vi "Trauma Box Controller.vi"() -> ()   [LabVIEW 2020]
uses:
  epl-vi-lib/Utility VIs/Buttons/KCheckmarkBoolean.ctl
  epl-vi-lib/Utility VIs/Controls/KBackground Gradient/KBackground Gradient.xctl
  Typedefs/TB-Parameters.ctl
  epl-vi-lib/Signal Synthesis VIs/Controls/Waveform XCtl/Waveform Enum.ctl
  Typedefs/TB-Slack State.ctl
  Typedefs/TB-State Enum.ctl
  <vilib>/Analysis/baseanly.llb/Mean (DBL).vi
  <vilib>/Analysis/5stat.llb/RMS (DBL).vi
  epl-vi-lib/Utility VIs/Math VIs/Linear to dB (scalar).vi
  epl-vi-lib/Connection VIs/Connection Manager.vi
  <vilib>/Analysis/NI_AALPro.lvlib
  <vilib>/Analysis/NI_AALBase.lvlib
  <vilib>/gmath/NI_Gmath.lvlib
panel:
  out "Exposure":errorcluster
  out "Crown":errorcluster
  in  "Waveform":u16(ring)=2 items=["Noise"=2, "File"=4, "Tone"=1]
  in  "dB SPL":dbl=100.0
  in  "Duration (min)":dbl=120.0
  in  "Tab Control":enum32{"Tone", "Noise", "File"}(tab)
  in  "Frequency (kHz)":dbl=8.0
  in  "High cutoff (kHz)":dbl=16.0
  in  "Low cutoff (kHz)":dbl=8.0
  in  "refWAV":path caption="Ref"
  in  "WAVfile":path
  in  "Cal Log":path=path "C:/Data/Trauma Box/Trauma Box Calibration Log.txt"
  out "Pistonphone Factor":dbl=102.0 caption="Calibrator Voltage\n(dB rms re 1 uV)"
  in  "B&K Mic Gain":dbl=20.0
  in  "Display":enum32{"Page 1", "Page 2"}(tab)
  out "ma":dbl=99.37258874088361 caption="average" format="%.1f"
  out "Starts":i32
  out "Overload 2":bool caption="Overload"
  in  "Fine Control":dbl(slide) caption="Fine Adjust (dB)" scale=0.0..1.0
  out "Spectrum":waveform(dbl)(graph)
  out "Waveform":waveform(dbl)(graph)
  out "dB SPL rms":dbl=99.37258874088361 format="%.2f"
  out "Gauge":dbl(knob)=99.37258874088361 scale=80.0..130.0
  out "Elapsed time":string
  out "SPL History":cluster{dbl[], dbl[]}[](graph)
  out "Expected":string="Expected value = 102"
  in  "micCorrFile":path
  in  "Use mic correction":T1 caption="Apply mic frequency correction (if you're unsure, then no)"
  out "Calibration Log":string[][](table)
  out "Overload":bool
  out "Calibrator Voltage\n(dB rms re 1 uV)":dbl=-inf
  out "Pistonphone\nWaveform":dbl[](graph)
  in  "Wizard":T2(tab)
  in  "START":bool
  in  "EXIT":bool
  in  "Use previous":bool
  in  "Remeasure":bool
  in  "Pistonphone measure":bool
  in  "Next":bool
  in  "To Crown adjust":bool
  in  "Start Crown":bool
  in  "Stop Crown":bool
  in  "Start Trauma":bool
  in  "Stop Trauma":bool
  in  "Finished":bool
  in  "User ID":string
  in  "Gradient":dbl(xcontrol)
  # "dB SPL"
  # "Press START to begin\nPress EXIT to quit"
  # "Step 1 Pistonphone correction"
  # "Step 1 Pistonphone correction\n    \n--Put ref mic into pistonphone\n--Make sure B&K gain is correct"
  # "Step 2 Put microphone in cage. It's going to get loud! Close the booth door before continuing."
  # "Step 3 Adjust amplifier until SPL is correct, then hit \"Stop\" button:"
  # "Step 4: Noise Exposure\n1. Put animal(s) in cage\n2. Set duration,\n3. Press START"
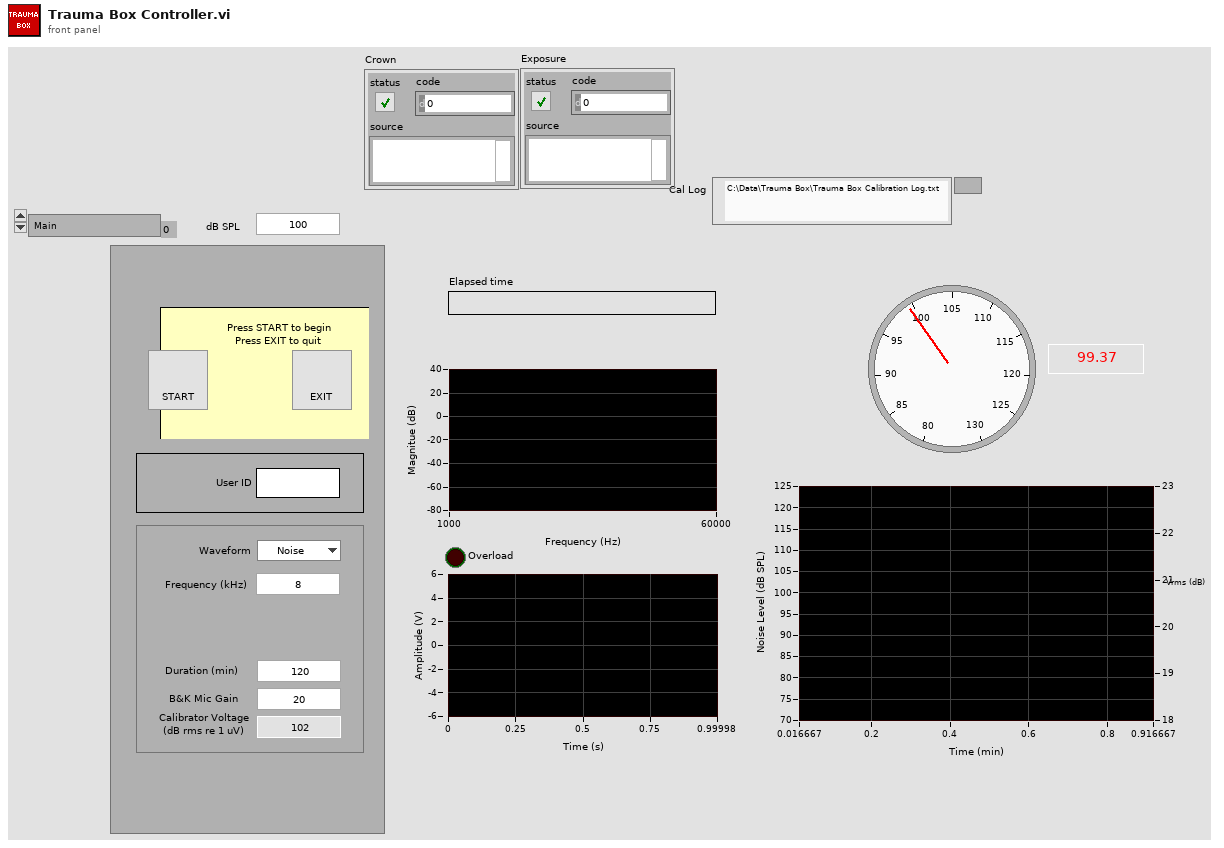
[diagram p1: front panel]
types:
  T1 = typedef "KCheckmarkBoolean.ctl" = bool
  T2 = enum32{"Main", "Pistonphone query", "Pistonphone measure", "Mic in cage", "Adjust Crown", "Animal in cage"}
  T3 = typedef "TB-Parameters.ctl" = cluster{"Low cutoff (kHz)":dbl, "High cutoff (kHz)":dbl, "Duration (min)":dbl, "dB SPL":dbl, "Waveform":T4, "WAVfile":path, "refWav":path, "use mic correction":bool, "micCorrFile":path, "Pistonphone Level (dB SPL)":dbl, "Sampling rate (Hz)":dbl, "Buffer length (s)":dbl, "Stream mic":bool, "Fine adjust":cluster{"Max":dbl, "Min":dbl}, "Mic gain":dbl, "atten":dbl, "resol (Hz)":dbl, "navgs":i32, "Allow Slack":bool, "max starts":i32, "Freq (kHz)":dbl, "Tma (s)":dbl, "Streamed":cluster{"Num":i32, "Name":string}[], "Drive":string}
  T4 = typedef "Waveform Enum.ctl" = enum16{"OFF", "Tone", "Noise", "Pulse Train", "File", "FM Sweep", "Chirp Train", "Complex Tone", "FM Tone", "Moving Ripple"}
  T5 = typedef "TB-Slack State.ctl" = cluster{"access_token":string, "bot id":string, "users":cluster{"id":string, "always":bool}[], "chan id":string}
  T6 = cluster{bool, "Exposure parameters":T3, "Slack":T5}
  T7 = typedef "TB-State Enum.ctl" = enum16{"Main", "Pistonphone query", "Pistonphone measure", "Mic in cage", "Adjust Crown", "Animal in cage"}
  T8 = enum16{"arithmetic", "geometric", "harmonic", "trimmed", "median"}
  T9 = cluster{"notification":bool, "Exposure parameters":T3, "Slack":T5}
  T10 = typedef "TB-Runtime state.ctl" = cluster{"stimfile":T11, "stream mic?":bool, "Fs":dbl, "ID":string, "micCorr":dbl[], "navg":i32, "r2sum":dbl[], "expose":bool, "spectra/frame":i32, "pts/spectra":i32, "nacq":i32, "init error":bool, "max starts":i32, "num starts":i32, "Setup":T12, "toneIndex":i32, "LastN":dbl[], "fine":dbl, "imic":i32, "stream":refnum<file>, "names":string[]}
  T11 = typedef "Sound File Refnum.ctl" = refnum<file>
  T12 = typedef "TB-Setup Log.ctl" = cluster{"Pistonphone factor":dbl, "Fine adjust":dbl, "Actual dB SPL":dbl, "Freq":dbl[], "Mag":dbl[]}
  T13 = typedef "TB-Stimulus State.ctl" = cluster{"filelen":i32, "stimfile":T11, "stimfile?":bool, "Fs":dbl, "Npts":i32, "stimfileend":bool, "atten":dbl, "AO":i32[]}
  T14 = typedef "Waveform XCtl.xctl/Waveform Data.ctl" = cluster{"Type":T4, "Tone":T15, "Pulse Train":T16, "Noise":T19, "File":T20, "FMSweep":T21, "Chirp Train":T22, "Complex Tone":cluster{"Params":T24, "Data":T26}, "Moving Ripple":T27}
  T15 = typedef "Tone Params.ctl" = cluster{"Frequency (kHz)":dbl, "Last Freq":dbl, "Last Phase":dbl}
  T16 = typedef "Pulse Train Params.ctl" = cluster{"Pulse width (us)":dbl, "Pulse rate (Hz)":dbl, "Gap (ms)":dbl, "Polarity":T17, "PT State":T18, "Asynch":bool}
  T17 = typedef "Pulse Polarity.ctl" = enum16{"POS", "NEG", "POS-NEG", "NEG-POS"}
  T18 = typedef "PT-Continuous State.ctl" = cluster{"Template":dbl[], "Nperiod":i32, "Index":i32, "Pulse Rate (Hz)":dbl, "Phase (cycles)":dbl, "Noff":i32}
  T19 = typedef "Noise Params.ctl" = cluster{"InvFilt":bool, "Noise":dbl[], "CurPt":i32, "Aweight":bool, "Seed":i32, "afile":path}
  T20 = typedef "StimFile-Params.ctl" = cluster{"Filename":path, "Signal":dbl[], "Channel":i32, "stream":bool, "offset":i32, "nreps":i32, "loops":i32, "Randomize":bool, "order":i32[], "Seed":i32, "Tokens":i32}
  T21 = typedef "FM Sweep Params.ctl" = cluster{"Rate (oct/s)":dbl, "Fmin (Hz)":dbl, "Fmax (Hz)":dbl, "Ramp (ms)":dbl, "Linear":bool}
  T22 = typedef "Chirp Train.ctl" = cluster{"Params":T23, "Data":cluster{"WF":dbl[]}}
  T23 = typedef "Chirp Train Params.ctl" = cluster{"Fmin (kHz)":dbl, "Fmax (kHz)":dbl, "Compensate":bool, "Duration (ms)":dbl}
  T24 = typedef "CT-Params.ctl" = cluster{"F0 (Hz)":dbl, "Band":cluster{"Flow (Hz)":dbl, "Fhigh (Hz)":dbl}, "Phase":T25, "Min F0 (Hz)":dbl, "Max F0 (Hz)":dbl, "ContinRandPhase":bool, "Max peak factor":dbl, "Max mod depth":dbl, "MinHarmNum":i32, "MaxHarmNum":i32, "Level Mode":enum16{"per component", "overall rms"}, "% jitter":dbl}
  T25 = typedef "CT-Phase Enum.ctl" = enum16{"Cosine", "Random", "Alternating"}
  T26 = typedef "CT-Runtime Data.ctl" = cluster{"Ncomp":i32, "MinHarm":i32, "Phase":dbl[], "Amplitude":dbl[], "Npts/frame":i32, "Last F0":dbl, "Fmin":dbl, "Fmax":dbl, "Lslope":dbl, "randphase":bool, "overall rms":bool, "fmult":dbl[], "jittered":bool}
  T27 = typedef "Moving Ripple.ctl" = cluster{"Params":T28, "Data":T29}
  T28 = typedef "Moving Ripple.Params.ctl" = cluster{"Fmin":dbl, "Fmax":dbl, "Density":dbl, "Velocity":dbl, "Depth":dbl, "Phase":dbl, "Comp/oct":i32}
  T29 = typedef "Moving Ripple.Data.ctl" = cluster{"Freq":dbl[], "A":dbl[], "phase":dbl[], "Phase":dbl}
  T30 = typedef "Filter XCtl.xctl/Filter Data.ctl" = cluster{"CF (kHz)":dbl, "BW (kHz)":dbl, "IIR Filter Cluster":cluster{"filter structure":enum32{"IIR 2nd Order", "IIR 4th Order"}, "Reverse Coefficients":dbl[], "Forward Coefficients":dbl[]}, "Final Filter State":dbl[], "Scale Factor":dbl, "Final Filter State 2":dbl[], "Quadrature":bool, "Type":enum16{"Lowpass", "Highpass", "Bandpass", "Bandstop", "OFF"}}
  T31 = typedef "Gate Control.xctl/Gate Data.ctl" = cluster{"Active":bool, "Delay (ms)":dbl, "Width (ms)":dbl, "Ramp (ms)":dbl}
  T32 = typedef "Level XCtl.xctl/Level Data.ctl" = cluster{"Level":dbl, "Units":T33, "Max":dbl, "Multiplier":dbl, "Cal File":path, "Cal":cluster{"Freq (Hz)":dbl[], "Mag (dB SPL)":dbl[], "Phase (deg)":dbl[]}}
  T33 = typedef "Level Units.ctl" = enum16{"dB atten", "dB SPL", "dB re 1 Vrms", "dB V/Hz½", "mW", "dB HL", "Volts", "dB mW"}
  T34 = cluster{"Waveform":T14, "Filter":T30, "Gate":T31, "Level":T32}
  T35 = typedef "TB-Log.ctl" = cluster{"Slack":T5, "entries":string[]}
  T36 = typedef "TB-Mic Queue.ctl" = refnum<queue>
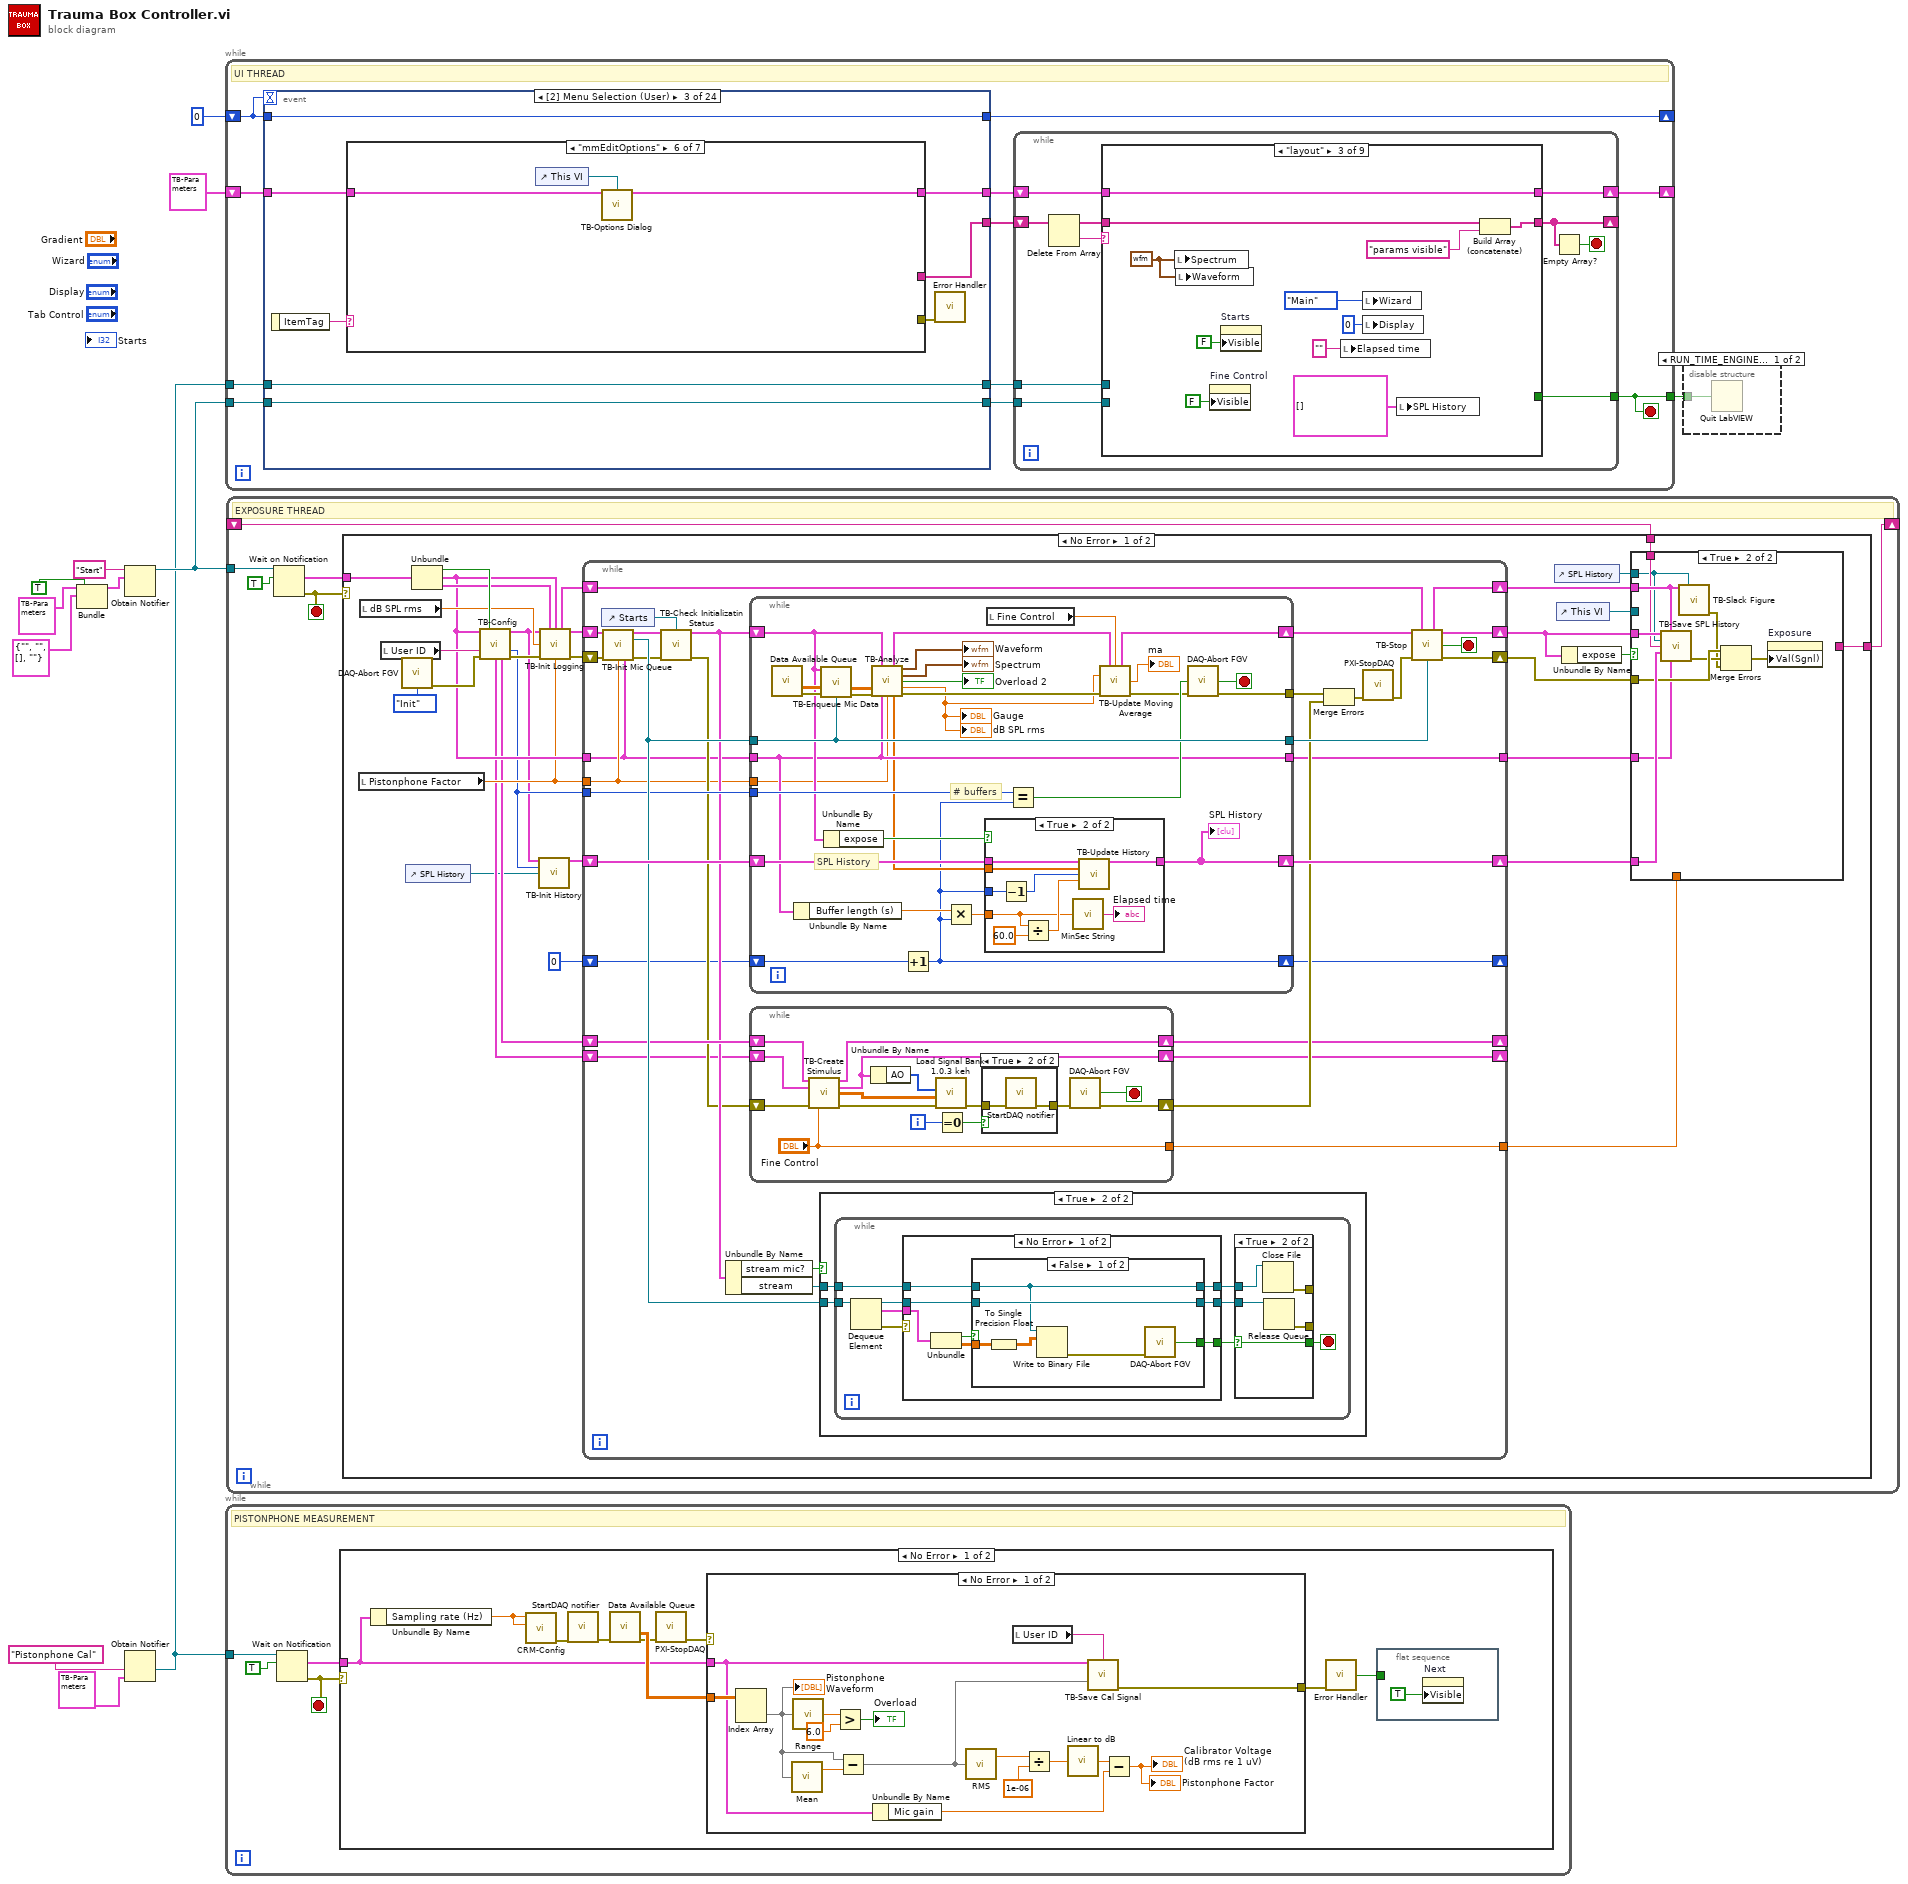
[diagram p0: block diagram]
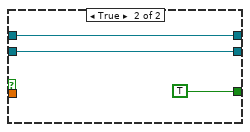
[diagram p6: hidden frame]
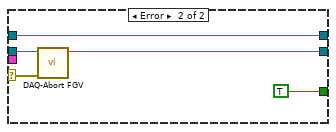
[diagram p7: hidden frame]
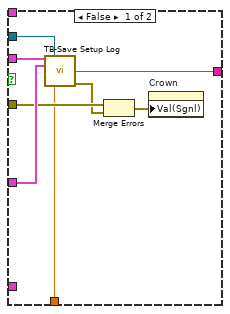
[diagram p8: hidden frame]
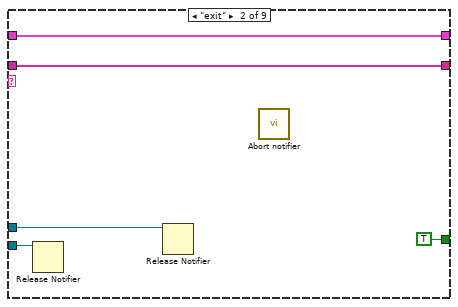
[diagram p11: hidden frame]
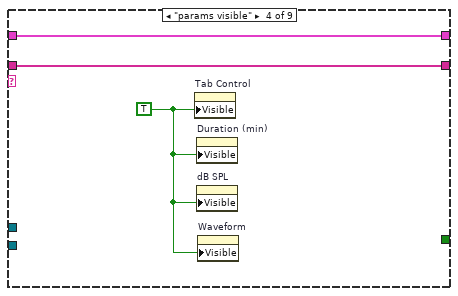
[diagram p12: hidden frame]
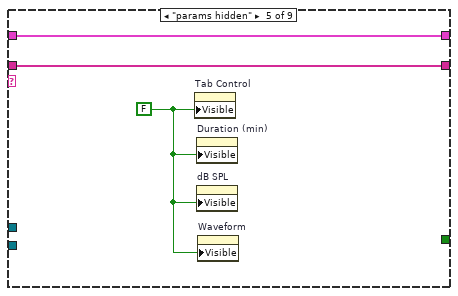
[diagram p13: hidden frame]
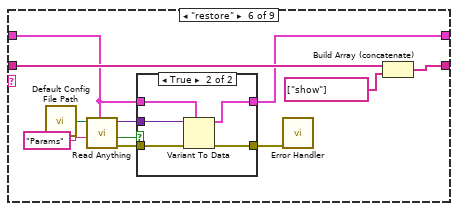
[diagram p14: hidden frame]
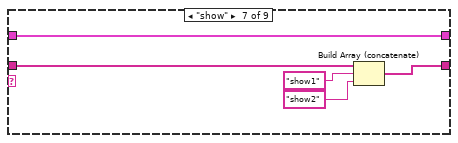
[diagram p16: hidden frame]
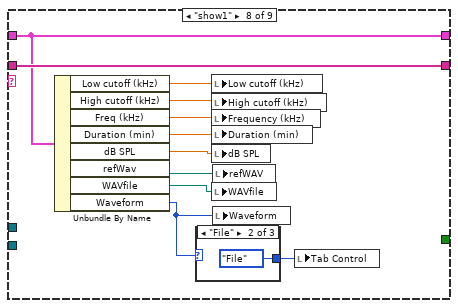
[diagram p17: hidden frame]
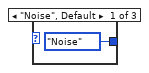
[diagram p18: hidden frame]
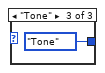
[diagram p19: hidden frame]
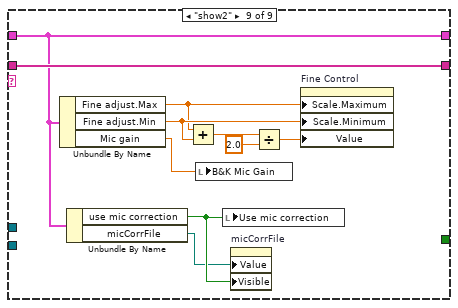
[diagram p20: hidden frame]
diagram:
  n1 = Bundle(TRUE, "Exposure parameters"=T3 {"Low cutoff (kHz)"=0.0, "High cutoff (kHz)"=0.0, "Duration (min)"=0.0, "dB SPL"=0.0, "Waveform"=enum."OFF", "WAVfile"=path "", "refWav"=path "", "use mic correction"=FALSE, "micCorrFile"=path "", "Pistonphone Level (dB SPL)"=0.0, "Sampling rate (Hz)"=0.0, "Buffer length (s)"=0.0, "Stream mic"=FALSE, "Fine adjust"={"Max"=0.0, "Min"=0.0}, "Mic gain"=0.0, "atten"=0.0, "resol (Hz)"=0.0, "navgs"=0, "Allow Slack"=FALSE, "max starts"=0, "Freq (kHz)"=8.0, "Tma (s)"=0.0, "Streamed"=[], "Drive"=""}, "Slack"=T5 {"access_token"="", "bot id"="", "users"=[], "chan id"=""}) -> (w4:T6)  [unwired: 1 in]
  n2 = Obtain Notifier(name (unnamed)="Start", notification data type=w4) -> (notifier out=w12:refnum<notifier>)  [unwired: 2 in, 2 out]
  n3 = Obtain Notifier(name (unnamed)="Pistonphone Cal", notification data type=T3 {"Low cutoff (kHz)"=114.0, "High cutoff (kHz)"=100000.0, "Duration (min)"=1.0, "dB SPL"=100.0, "Waveform"=enum."Noise", "WAVfile"=path "", "refWav"=path "", "use mic correction"=FALSE, "micCorrFile"=path "", "Pistonphone Level (dB SPL)"=0.0, "Sampling rate (Hz)"=0.0, "Buffer length (s)"=0.0, "Stream mic"=FALSE, "Fine adjust"={"Max"=0.0, "Min"=0.0}, "Mic gain"=0.0, "atten"=0.0, "resol (Hz)"=0.0, "navgs"=0, "Allow Slack"=FALSE, "max starts"=0, "Freq (kHz)"=8.0, "Tma (s)"=0.0, "Streamed"=[], "Drive"=""} ("Exposure parameters")) -> (notifier out=w8:refnum<notifier>)  [unwired: 2 in, 2 out]
  n4 = while {
    tunnel: w12 -> [w23]
    shift-right: [w22] -> _
    shift-left: 0 -> [w19]
    tunnel: w8 -> [w21]
    tunnel: [w13] -> w7
    shift-right: [w14] -> _
    shift-left: T3 {"Low cutoff (kHz)"=8.0, "High cutoff (kHz)"=16.0, "Duration (min)"=120.0, "dB SPL"=100.0, "Waveform"=enum."Noise", "WAVfile"=path "", "refWav"=path "", "use mic correction"=FALSE, "micCorrFile"=path "", "Pistonphone Level (dB SPL)"=114.0, "Sampling rate (Hz)"=100000.0, "Buffer length (s)"=1.0, "Stream mic"=FALSE, "Fine adjust"={"Max"=0.0, "Min"=0.0}, "Mic gain"=0.0, "atten"=0.0, "resol (Hz)"=0.0, "navgs"=0, "Allow Slack"=FALSE, "max starts"=3, "Freq (kHz)"=8.0, "Tma (s)"=0.0, "Streamed"=[], "Drive"=""} ("Exposure parameters") -> [w20]
    stop <- w13 stop-if-true
    # "UI THREAD"
    n5 = event shown="[2] Menu Selection (User)" {
      selector: _ -> [_ _ _ _ _ _ _ _ _ _ _ _ _ _ _ _ _ _ _ _ _ _ _ _]
      dyn-events: _ -> [_ _ _ _ _ _ _ _ _ _ _ _ _ _ _ _ _ _ _ _ _ _ _ _]
      timeout: w19 -> [_ _ _ _ _ _ _ _ _ _ _ _ _ _ _ _ _ _ _ _ _ _ _ _]
      tunnel: w23 -> [_ w139 w146 _ _ _ _ _ _ _ _ _ _ _ _ w248 w256 _ w291 _ _ w312 _ _]
      tunnel: [_ w139 w146 _ _ _ _ _ _ _ _ _ _ _ _ _ _ _ _ _ _ w312 _ _] -> w16
      tunnel: [-1 w142 w150 w178 w184 w190 w193 w198 w206 w207 w212 w219 w223 w229 w232 w241 w252 w264 w274 w303 w305 w309 w316 w320] -> w22
      tunnel: w21 -> [_ w140 w147 _ _ _ _ _ _ _ _ _ _ w230 _ _ _ _ _ _ _ w311 _ _]
      tunnel: [_ w140 w147 _ _ _ _ _ _ _ _ _ _ _ _ _ _ _ _ _ _ w311 _ _] -> w17
      tunnel: [w109 w143 w148 w179 w187 w191 w196 w201 w204 w210 w213 w220 w224 w228 w233 w238 w253 w265 w272 w304 w306 w310 w315 w319] -> w15
      tunnel: w20 -> [w109 w143 w151 w180 w188 w192 w197 w202 w205 w211 w213 w220 w224 w228 w233 w238 w253 w265 w272 w304 w306 w310 w315 w319]
      tunnel: w19 -> [_ w142 w150 w178 w184 w190 w193 w198 w206 w207 w212 w219 w223 w229 w232 w241 w252 w264 w274 w303 w305 w309 w316 w320]
      tunnel: [string[] ["restore", "layout"] string[] ["exit"] w149 _ _ _ _ _ _ _ _ _ string[] ["params hidden"] _ string[] ["params visible"] _ _ _ _ _ _ string[] ["exit"] _ _] -> w18
      event Timeout {
        n6 = event-data() -> ()  [unwired: 1 in, 1 out]
        n7 = call "SGDA-Initialize Hardware.vi"() -> ("error out"=w110:errorcluster)  [unwired: 14 in, 1 out]
        n8 = call "Error Handler.vi"("error in (no error)"=w110) -> ()  [unwired: 13 in, 2 out]
        n9 = Read from Text File(file (use dialog)="Cal Log") -> (text=w112:string, error out=w113:errorcluster)  [unwired: 3 in, 2 out]
        n10 = case shown="No Error" w113 {
          tunnel: w112 -> [w129 _]
          tunnel: [w124 _] -> w111
          tunnel: [w116 102.0] -> w107
          frame No Error {
            n11 = Spreadsheet String To Array(format string="%s", spreadsheet string=w129, array type (2D Dbl)=string[][] []) -> (array=w126:string[][])  [unwired: 1 in]
            n12 = Transpose 2D Array(2D array=w126) -> (transposed array=w123:string[][])
            n13 = Index Array(array=w123, index (row)=2) -> (element=w121:string[])  [unwired: 1 in]
            n14 = for {
              tunnel: w123 -> [w137] mode=indexing
              tunnel: [w136] -> w125 mode=indexing
              n15 = Reverse 1D Array(array=w137) -> (reversed array=w136:string[])
            }
            n16 = for {
              tunnel: w121 -> [w135] mode=indexing
              tunnel: "%g" ("format string") -> [w134]
              tunnel: [w132] -> w118 mode=indexing if=w130
              tunnel: nan ("default (0 dbl)") -> [w133]
              n17 = Scan Value(string=w135, format string=w134, default (0 dbl)=w133) -> (value=w132:dbl)  [unwired: 1 out]
              n18 = Not A Number/Path/Refnum?(number/path/refnum=w132) -> (NaN/Path/Refnum?=w131:bool)
              n19 = Not(x=w131) -> (.not. x?=w130:bool)
            }
            n20 = Transpose 2D Array(2D array=w125) -> (transposed array=w124:string[][])
            n21 = call <vilib>:"Measures of Mean.vi"("type"=T8."median", "x array"=w118) -> ("mean value"=w116:dbl)  [unwired: 8 in, 1 out]
          }
          frame Error {
          }
        }
        "Calibration Log" <- w111
        n22 = local write "Pistonphone Factor"(w107) -> ()
        n23 = Format Into String(format string="Expected value = %d", w107) -> (resulting string=→"Expected":string)  [unwired: 2 in, 1 out]
      }
      event Panel Close? {
        n24 = event-data() -> ()  [unwired: 1 in, 1 out]
        n25 = event-data("Discard?"=TRUE) -> ()  [unwired: 1 in, 1 out]
      }
      event Menu Selection (User) {
        n26 = event-data() -> ("ItemTag"=w152:string)  [unwired: 1 in]
        n27 = case shown="\"mmEditOptions\"" w152 {
          tunnel: [_ _ w161 _ _ _ _] -> w145
          tunnel: w151 -> [w153 w154 w158 w167 w169 w171 w173]
          tunnel: [w153 w154 w157 w167 w169 w172 w173] -> w148
          tunnel: [_ string[] ["restore"] _ string[] ["restore", "layout"] string[] ["exit"] _ _] -> w149
          frame "", Default {
          }
          frame "mmFileRestore" {
          }
          frame "mmFileSave" {
            n28 = property on="Fine Control" class="Slide (strict)"() -> ("Scale.Maximum"=w160:dbl, "Scale.Minimum"=w159:dbl)  [unwired: 2 in, 2 out]
            n29 = Bundle By Name(cluster=w158, "Fine adjust.Max"=w160, "Fine adjust.Min"=w159) -> (w157:T3)
            n30 = call "Default Config File Path.vi"() -> ("Default config file name"=w163:path)
            n31 = call "Write Anything.vi"("Section Name (Name of \"Anything\")"="Params" ("Section Name (Name of \"Anything\")"), "Anything"=w157, "Path (dialog)"=w163) -> ("Error Out"=w162:errorcluster)  [unwired: 7 in, 1 out]
            n32 = case shown="No Error" w162 {
              selector: w162 -> [_ w165]
              tunnel: [_ w165] -> w161
              frame No Error {
                n33 = One Button Dialog(message="Defaults saved.") -> ()  [unwired: 1 in, 1 out]
              }
              frame Error {
              }
            }
          }
          frame "mmFileRestart" {
          }
          frame "mmFileExit" {
          }
          frame "mmEditOptions" {
            n34 = control-ref of="This VI"() -> (w170:refnum<vi>)
            n35 = call "TB-Options Dialog.vi"("Parameters in"=w171, "Parent VI"=w170) -> ("Parameters out"=w172:T3)  [unwired: 12 in, 1 out]
          }
          frame "mmEditConfig" {
            n36 = One Button Dialog(message="Note: Trauma Box Controller sends noise to the \"Background\" output, and records from the microphone using the \"Cal Mic\" input.", button name ("OK")="Continue") -> ()  [unwired: 1 out]
            n37 = call-by-ref "?"() -> ()  [unwired: 14 in, 2 out]
          }
        }
        n38 = call "Error Handler.vi"("error in (no error)"=w145) -> ()  [unwired: 13 in, 2 out]
      }
      event "Waveform": Value Change {
        n39 = event-data() -> ()  [unwired: 1 in, 1 out]
        n40 = case shown="1" "Waveform" {
          tunnel: [enum32{"Tone", "Noise", "File"}."Noise" ("Tab Control") enum32{"Tone", "Noise", "File"}."File" ("Tab Control") enum32{"Tone", "Noise", "File"}."Tone" ("Tab Control")] -> w177
          frame 2, Default {
          }
          frame 4 {
          }
          frame 1 {
          }
        }
        n41 = local write "Tab Control"(w177) -> ()
        n42 = Bundle By Name(cluster=w180, "Waveform"="Waveform") -> (w179:T3)
      }
      event "Low cutoff (kHz)", "High cutoff (kHz)": Value Change {
        n43 = event-data() -> ()  [unwired: 1 in, 1 out]
        n44 = Bundle By Name(cluster=w188, "Low cutoff (kHz)"="Low cutoff (kHz)", "High cutoff (kHz)"="High cutoff (kHz)") -> (w187:T3)
      }
      event "Frequency (kHz)": Value Change {
        n45 = event-data() -> ()  [unwired: 1 in, 1 out]
        n46 = Bundle By Name(cluster=w192, "Freq (kHz)"="Frequency (kHz)") -> (w191:T3)
      }
      event "WAVfile", "refWAV": Value Change {
        n47 = event-data() -> ()  [unwired: 1 in, 1 out]
        n48 = Bundle By Name(cluster=w197, "WAVfile"="WAVfile", "refWav"="refWAV") -> (w196:T3)
      }
      event "micCorrFile": Value Change {
        n49 = event-data() -> ()  [unwired: 1 in, 1 out]
        n50 = Bundle By Name(cluster=w202, "use mic correction"="Use mic correction", "micCorrFile"="micCorrFile") -> (w201:T3)
        n51 = property on="micCorrFile" class="Path"("Visible"="Use mic correction") -> ()  [unwired: 2 in, 2 out]
      }
      event "B&K Mic Gain": Value Change {
        n52 = event-data() -> ()  [unwired: 1 in, 1 out]
        n53 = Bundle By Name(cluster=w205, "Mic gain"="B&K Mic Gain") -> (w204:T3)
      }
      event "Duration (min)", "dB SPL": Value Change {
        n54 = event-data() -> ()  [unwired: 1 in, 1 out]
        n55 = Bundle By Name(cluster=w211, "Duration (min)"="Duration (min)", "dB SPL"="dB SPL") -> (w210:T3)
      }
      event "START": Value Change {
        n56 = event-data() -> ()  [unwired: 1 in, 1 out]
        n57 = Empty String/Path?(string/path="User ID") -> (empty?=w214:bool)
        n58 = case shown="False" w214 {
          frame False {
            n59 = property on="Starts" class="DigNum (strict)"("Visible"=FALSE) -> ()  [unwired: 2 in, 2 out]
            n60 = local write "Wizard"(TB-State_Enum."Pistonphone query" ("State")) -> ()
          }
          frame True {
            n61 = One Button Dialog(message="Please enter a User ID (for bookkeeping purposes).") -> ()  [unwired: 1 in, 1 out]
          }
        }
      }
      event "Use previous": Value Change {
        n62 = event-data() -> ()  [unwired: 1 in, 1 out]
        n63 = local write "Wizard"(TB-State_Enum."Mic in cage" ("State")) -> ()
      }
      event "Remeasure": Value Change {
        n64 = event-data() -> ()  [unwired: 1 in, 1 out]
        n65 = property on="Next" class="Bool"("Visible"=FALSE) -> ()  [unwired: 2 in, 2 out]
        n66 = local write "Display"(1) -> ()
        n67 = local write "Wizard"(TB-State_Enum."Pistonphone measure" ("State")) -> ()
      }
      event "Pistonphone measure": Value Change {
        n68 = event-data() -> ()  [unwired: 1 in, 1 out]
        n69 = Send Notification(notification=w228, notifier=w230) -> ()  [unwired: 1 in, 2 out]
      }
      event "Next": Value Change {
        n70 = event-data() -> ()  [unwired: 1 in, 1 out]
        n71 = local write "Wizard"(TB-State_Enum."Mic in cage" ("State")) -> ()
        n72 = local write "Display"(0) -> ()
      }
      event "To Crown adjust": Value Change {
        n73 = event-data() -> ()  [unwired: 1 in, 1 out]
        n74 = property on="Fine Control" class="Slide (strict)"("Visible"=TRUE, "Value"=0.0 ("Fine Control")) -> (error out=w243:errorcluster)  [unwired: 2 in, 1 out]
        n75 = local write "Elapsed time"("" ("Elapsed time")) -> ()
        n76 = local write "Wizard"(TB-State_Enum."Adjust Crown" ("State")) -> ()
        n77 = Bundle("notification"=FALSE, "Exposure parameters"=w238, "Slack"=T5 {"access_token"="", "bot id"="", "users"=[], "chan id"=""}) -> (w240:T9)  [unwired: 1 in]
        n78 = Send Notification(notification=w240, notifier=w248, error in (no error)=w243) -> ()  [unwired: 2 out]
        n79 = property on="Start Crown" class="Bool"("Visible"=FALSE) -> ()  [unwired: 2 in, 2 out]
        n80 = Unbundle By Name(w238) -> ("Tma (s)"=w237:dbl)
        n81 = Greater Than 0?(x=w237) -> (x > 0?=w236:bool)
        n82 = property on="ma" class="DigNum (strict)"("Visible"=w236) -> ()  [unwired: 2 in, 2 out]
      }
      event "Start Crown": Value Change {
        n83 = event-data() -> ()  [unwired: 1 in, 1 out]
        n84 = while {
          tunnel: w256 -> [w262]
          tunnel: [w258] -> w255
          stop <- w260 stop-if-true
          n85 = Get Notifier Status(notifier=w262) -> (notifier out=w258:refnum<notifier>, # waiting=w261:i32)  [unwired: 1 in, 3 out]
          n86 = Wait (ms)(milliseconds to wait=u32 250) -> ()  [unwired: 1 out]
          n87 = Greater Than 0?(x=w261) -> (x > 0?=w260:bool)
        }
        n88 = Bundle("notification"=FALSE, "Exposure parameters"=w253, "Slack"=T5 {"access_token"="", "bot id"="", "users"=[], "chan id"=""}) -> (w251:T9)  [unwired: 1 in]
        n89 = Send Notification(notification=w251, notifier=w255) -> ()  [unwired: 1 in, 2 out]
        n90 = property on="Start Crown" class="Bool"("Visible"=FALSE) -> ()  [unwired: 2 in, 2 out]
      }
      event "Stop Crown": Value Change {
        w266 = TRUE ("Visible")
        n91 = event-data() -> ()  [unwired: 1 in, 1 out]
        n92 = local write "Wizard"(TB-State_Enum."Animal in cage" ("State")) -> ()
        n93 = property on="Start Trauma" class="Bool"("Visible"=w266) -> ()  [unwired: 2 in, 2 out]
        n94 = property on="Stop Trauma" class="Bool"("Visible"=w266) -> ()  [unwired: 2 in, 2 out]
        n95 = call "DAQ-Abort FGV.vi"("Action"=enum16{"Default", "Init", "Abort", "1st error"}."Abort") -> ()  [unwired: 12 in, 3 out]
      }
      event "Start Trauma": Value Change {
        n96 = event-data() -> ("CtlRef"=w269:refnum<vi>)  [unwired: 1 in]
        n97 = local read "Pistonphone Factor"() -> (w285:dbl)
        n98 = Get Date/Time In Seconds() -> (seconds since 1Jan1904=w286:timestamp)
        n99 = local read "User ID"() -> (w287:string)
        n100 = local read "Cal Log"() -> (w277:path)
        n101 = Get Date/Time String(seconds (now)=w286) -> (date string=w284:string)  [unwired: 2 in, 1 out]
        n102 = Strip Path(path=w277) -> (stripped path=w279:path)  [unwired: 1 out]
        n103 = property on="Start Trauma" class="Bool"("Visible"=FALSE) -> ()  [unwired: 2 in, 2 out]
        n104 = call "FileIO-File or Folder Exists.vi"("path"=w279) -> ("Directory?"=w278:bool, "dup path"=w276:path)  [unwired: 7 in, 2 out]
        n105 = Format Into String(format string="%s\t%s\t%.2f\n", w287, w284, w285) -> (resulting string=w288:string)  [unwired: 2 in, 1 out]
        n106 = case shown="False" w278 {
          tunnel: w276 -> [w296 _]
          tunnel: [w295 _] -> w275
          frame False {
            n107 = Create Folder(path (use dialog)=w296) -> (error out=w295:errorcluster)  [unwired: 2 in, 2 out]
          }
          frame True {
          }
        }
        n108 = Unbundle By Name(w272) -> ("Duration (min)"=w281:dbl)
        n109 = call "Append to Text File.vi"("file path"=w277, "text"=w288, "error in (no error)"=w275) -> ("error out"=w282:errorcluster)  [unwired: 11 in, 1 out]
        n110 = property on="SPL History" class="XYGraph (strict)"(error in=w282, "XScale.Maximum"=w281) -> (error out=w283:errorcluster)  [unwired: 1 in, 1 out]
        n111 = Unbundle By Name(w272) -> ("Allow Slack"=w270:bool)
        n112 = property on="ma" class="DigNum (strict)"("Visible"=FALSE) -> ()  [unwired: 2 in, 2 out]
        n113 = while {
          tunnel: w291 -> [w301]
          tunnel: [w297] -> w292
          tunnel: w283 -> [_]
          stop <- w299 stop-if-true
          n114 = Wait (ms)(milliseconds to wait=u32 250) -> ()  [unwired: 1 out]
          n115 = Get Notifier Status(notifier=w301) -> (notifier out=w297:refnum<notifier>, # waiting=w300:i32)  [unwired: 1 in, 3 out]
          n116 = Greater Than 0?(x=w300) -> (x > 0?=w299:bool)
        }
        n117 = call "TB-Init Slack.vi"("Allow Slack"=w270, "CtlRef"=w269) -> ("Slack"=w271:T5)  [unwired: 13 in]
        n118 = property on="Stop Trauma" class="Bool"("Visible"=TRUE) -> ()  [unwired: 2 in, 2 out]
        n119 = Bundle("notification"=TRUE, "Exposure parameters"=w272, "Slack"=w271) -> (w273:T9)  [unwired: 1 in]
        n120 = property on="Fine Control" class="Slide (strict)"("Visible"=FALSE) -> ()  [unwired: 2 in, 2 out]
        n121 = Send Notification(notification=w273, notifier=w292) -> ()  [unwired: 1 in, 2 out]
      }
      event "Stop Trauma": Value Change {
        n122 = event-data() -> ()  [unwired: 1 in, 1 out]
        n123 = call "DAQ-Abort FGV.vi"("Action"=enum16{"Default", "Init", "Abort", "1st error"}."Abort") -> ()  [unwired: 12 in, 3 out]
      }
      event "Finished": Value Change {
        n124 = event-data() -> ()  [unwired: 1 in, 1 out]
        n125 = local write "Wizard"(TB-State_Enum."Main" ("State")) -> ()
      }
      event "EXIT": Value Change {
        n126 = event-data() -> ()  [unwired: 1 in, 1 out]
      }
      event "Crown": Value Change {
        n127 = event-data() -> ("NewVal"=w314:errorcluster, "NewVal.status"=w313:bool)  [unwired: 1 in]
        n128 = property on="Start Crown" class="Bool"("Visible"=w313) -> ()  [unwired: 2 in, 2 out]
        n129 = call "Error Handler.vi"("error in (no error)"=w314) -> ()  [unwired: 13 in, 2 out]
      }
      event "Exposure": Value Change {
        n130 = event-data() -> ("NewVal"=w317:errorcluster)  [unwired: 1 in]
        n131 = call "Error Handler.vi"("error in (no error)"=w317) -> ()  [unwired: 13 in, 2 out]
        n132 = property on="Stop Trauma" class="Bool"("Visible"=FALSE) -> ()  [unwired: 2 in, 2 out]
      }
    }
    n133 = while {
      shift-right: [w30] -> _
      shift-left: w18 -> [w33]
      tunnel: w17 -> [w28]
      tunnel: w16 -> [w27]
      shift-right: [w25] -> w14
      shift-left: w15 -> [w26]
      tunnel: [w24] -> w13
      stop <- w29 stop-if-true
      n134 = Delete From Array(array=w33) -> (deleted portion=w31:string, array with subset deleted=w32:string[])  [unwired: 2 in]
      n135 = case shown="\"layout\"" w31 {
        tunnel: w32 -> [w35 w40 w51 w54 w57 w68 w80 w91 w104]
        tunnel: [w35 w40 w44 w54 w57 w59 w78 w91 w104] -> w30
        tunnel: w28 -> [_ w39 _ _ _ _ _ _ _]
        tunnel: w27 -> [_ w38 _ _ _ _ _ _ _]
        tunnel: w26 -> [w34 w37 w50 w53 w56 w60 w79 w84 w95]
        tunnel: [w34 w37 w50 w53 w56 w62 w79 w84 w95] -> w25
        tunnel: [_ TRUE _ _ _ _ _ _ _] -> w24
        frame "", Default {
        }
        frame "exit" {
          n136 = Release Notifier(notifier=w38) -> ()  [unwired: 2 in, 3 out]
          n137 = Release Notifier(notifier=w39) -> ()  [unwired: 2 in, 3 out]
          n138 = call "Abort notifier.vi"() -> ()  [unwired: 6 in, 2 out]
        }
        frame "layout" {
          w49 = waveform(dbl) {"t0"=timestamp(0 s since 1904-01-01), "dt"=1.0, "Y"=[]} ("Spectrum")
          n139 = local write "Spectrum"(w49) -> ()
          n140 = local write "Waveform"(w49) -> ()
          n141 = property on="Fine Control" class="Slide (strict)"("Visible"=FALSE) -> ()  [unwired: 2 in, 2 out]
          n142 = property on="Starts" class="DigNum (strict)"("Visible"=FALSE) -> ()  [unwired: 2 in, 2 out]
          n143 = local write "Elapsed time"("") -> ()
          n144 = local write "Wizard"(TB-State_Enum."Main" ("State")) -> ()
          n145 = local write "Display"(0) -> ()
          n146 = local write "SPL History"(cluster{dbl[], dbl[]}[] [] ("SPL History")) -> ()
          n147 = Build Array (concatenate)(w51, "params visible") -> (w44:string[])
        }
        frame "params visible" {
          w52 = TRUE
          n148 = property on="Tab Control" class="TabCtl (strict)"("Visible"=w52) -> ()  [unwired: 2 in, 2 out]
          n149 = property on="Duration (min)" class="DigNum (strict)"("Visible"=w52) -> ()  [unwired: 2 in, 2 out]
          n150 = property on="dB SPL" class="DigNum (strict)"("Visible"=w52) -> ()  [unwired: 2 in, 2 out]
          n151 = property on="Waveform" class="Ring (strict)"("Visible"=w52) -> ()  [unwired: 2 in, 2 out]
        }
        frame "params hidden" {
          w55 = FALSE
          n152 = property on="Tab Control" class="TabCtl (strict)"("Visible"=w55) -> ()  [unwired: 2 in, 2 out]
          n153 = property on="Duration (min)" class="DigNum (strict)"("Visible"=w55) -> ()  [unwired: 2 in, 2 out]
          n154 = property on="dB SPL" class="DigNum (strict)"("Visible"=w55) -> ()  [unwired: 2 in, 2 out]
          n155 = property on="Waveform" class="Ring (strict)"("Visible"=w55) -> ()  [unwired: 2 in, 2 out]
        }
        frame "restore" {
          n156 = call "Default Config File Path.vi"() -> ("Default config file name"=w65:path)
          n157 = call "Read Anything.vi"("Type of Anything"=w60, "Section Name (Name of \"Type of Anything\")"="Params" ("Section Name (Name of \"Type of Anything\")"), "Path (dialog)"=w65) -> ("Error Out"=w63:errorcluster, "Found?"=w61:bool, "Anything"=w64:variant)  [unwired: 6 in]
          n158 = case shown="True" w61 {
            tunnel: [w69 w75] -> w66
            tunnel: w64 -> [_ w74]
            tunnel: w63 -> [w69 w73]
            tunnel: [w70 w72] -> w62
            tunnel: w60 -> [w70 w71]
            frame False {
            }
            frame True {
              n159 = Variant To Data(error in=w73, type=w71, Variant=w74) -> (data=w72:T3, error out=w75:errorcluster)
            }
          }
          n160 = call "Error Handler.vi"("error in (no error)"=w66) -> ()  [unwired: 13 in, 2 out]
          n161 = Build Array (concatenate)(w68, string[] ["show"]) -> (w59:string[])
        }
        frame "show" {
          n162 = Build Array (concatenate)(w80, "show1", "show2") -> (w78:string[])
        }
        frame "show1" {
          n163 = Unbundle By Name(w84) -> ("Low cutoff (kHz)"=w85:dbl, "High cutoff (kHz)"=w86:dbl, "Freq (kHz)"=w81:dbl, "Duration (min)"=w87:dbl, "dB SPL"=w88:dbl, "refWav"=w90:path, "WAVfile"=w89:path, "Waveform"=w83:T4)
          n164 = case shown="\"File\"" w83 {
            tunnel: [enum32{"Tone", "Noise", "File"}."Noise" ("Tab Control") enum32{"Tone", "Noise", "File"}."File" ("Tab Control") enum32{"Tone", "Noise", "File"}."Tone" ("Tab Control")] -> w82
            frame "Noise", Default {
            }
            frame "File" {
            }
            frame "Tone" {
            }
          }
          n165 = local write "Low cutoff (kHz)"(w85) -> ()
          n166 = local write "High cutoff (kHz)"(w86) -> ()
          n167 = local write "Frequency (kHz)"(w81) -> ()
          n168 = local write "Duration (min)"(w87) -> ()
          n169 = local write "dB SPL"(w88) -> ()
          n170 = local write "WAVfile"(w89) -> ()
          n171 = local write "refWAV"(w90) -> ()
          n172 = local write "Waveform"(w83) -> ()
          n173 = local write "Tab Control"(w82) -> ()
        }
        frame "show2" {
          n174 = Unbundle By Name(w95) -> ("Fine adjust.Max"=w99:dbl, "Fine adjust.Min"=w100:dbl, "Mic gain"=w103:dbl)
          n175 = Unbundle By Name(w95) -> ("use mic correction"=w97:bool, "micCorrFile"=w96:path)
          n176 = Add(x=w99, y=w100) -> (x+y=w98:dbl)
          n177 = local write "B&K Mic Gain"(w103) -> ()
          n178 = local write "Use mic correction"(w97) -> ()
          n179 = property on="micCorrFile" class="Path"("Value"=w96, "Visible"=w97) -> ()  [unwired: 2 in, 2 out]
          n180 = Divide(x=w98, y=2.0) -> (x/y=w101:dbl)
          n181 = property on="Fine Control" class="Slide (strict)"("Scale.Maximum"=w99, "Scale.Minimum"=w100, "Value"=w101) -> ()  [unwired: 2 in, 2 out]
        }
      }
      n182 = Empty Array?(array=w30) -> (empty?=w29:bool)
    }
  }
  n183 = while {
    tunnel: w8 -> [w323]
    stop <- w322 stop-if-true
    # "PISTONPHONE MEASUREMENT"
    n184 = Wait on Notification(notifier=w323, ignore previous (F)=TRUE) -> (notification=w321:T3, error out=w322:errorcluster)  [unwired: 2 in, 2 out]
    n185 = case shown="No Error" w322 {
      tunnel: w321 -> [w325 _]
      frame No Error {
        n186 = Unbundle By Name(w325) -> ("Sampling rate (Hz)"=w326:dbl)
        n187 = call "CRM-Config.vi"("Num AI pts"=w326, "Sampling Rate (Hz)"=w326) -> ("error out"=w333:errorcluster)  [unwired: 7 in, 2 out]
        n188 = call "StartDAQ notifier.vi"("error in (no error)"=w333) -> ("error out"=w332:errorcluster)  [unwired: 6 in]
        n189 = call "Data Available Queue.vi"("error in (no error)"=w332) -> ("AI Waveforms"=w331:dbl[][], "error out"=w330:errorcluster)  [unwired: 10 in, 3 out]
        n190 = call "PXI-StopDAQ.vi"("error in (no error)"=w330) -> ("error out"=w329:errorcluster)  [unwired: 6 in]
        n191 = case shown="No Error" w329 {
          selector: w329 -> [_ w350]
          tunnel: w331 -> [w349 _]
          tunnel: [w336 w350] -> w328
          tunnel: w325 -> [w335 _]
          frame No Error {
            n192 = Index Array(array=w349) -> (element=w345:dbl[])  [unwired: 2 in]
            "Pistonphone\nWaveform" <- w345
            n193 = call-poly <vilib>:"Mean.vi"("X"=w345) -> ("mean"=w344:dbl)  [unwired: 1 out]
            n194 = call "Range.vi"("Array"=w345) -> ("Range"=w348:dbl)
            n195 = Greater?(x=w348, y=6.0) -> (0:→"Overload":bool)
            n196 = Subtract(x=w345, y=w344) -> (x-y=w337:dbl[])
            n197 = Unbundle By Name(w335) -> ("Mic gain"=w334:dbl)
            n198 = call-poly <vilib>:"RMS.vi"("X"=w337) -> ("rms value"=w343:dbl)  [unwired: 1 out]
            n199 = local read "User ID"() -> (w338:string)
            n200 = Divide(x=w343, y=1e-06) -> (x/y=w341:dbl)
            n201 = call-poly "Linear to dB.vi"("Linear"=w341) -> ("dB"=w340:dbl)
            n202 = call "TB-Save Cal Signal.vi"("Params"=w335, "ID"=w338, "Mic signal"=w337) -> ("error out"=w336:errorcluster)  [unwired: 12 in]
            n203 = Subtract(x=w340, y=w334) -> (x-y=→"Calibrator Voltage\n(dB rms re 1 uV)" →"Pistonphone Factor":dbl)
          }
          frame Error {
          }
        }
        n204 = call "Error Handler.vi"("error in (no error)"=w328) -> ("error?"=w327:bool)  [unwired: 13 in, 1 out]
        n205 = flat-sequence {
          tunnel: w327 -> [_]
          frame #0 {
            n206 = property on="Next" class="Bool"("Visible"=TRUE) -> ()  [unwired: 2 in, 2 out]
          }
        }
      }
      frame Error {
      }
    }
  }
  n207 = while {
    tunnel: w12 -> [w356]
    shift-right: [w353] -> _
    shift-left: _ -> [w352]
    stop <- w355 stop-if-true
    # "EXPOSURE THREAD"
    n208 = Wait on Notification(notifier=w356, ignore previous (F)=TRUE) -> (notification=w354:T6, error out=w355:errorcluster)  [unwired: 2 in, 2 out]
    n209 = case shown="No Error" w355 {
      tunnel: w354 -> [w388 _]
      tunnel: [w365 _] -> w353
      tunnel: w352 -> [w364 _]
      frame No Error {
        n210 = local read "Pistonphone Factor"() -> (w368:dbl)
        n211 = local read "dB SPL rms"() -> (w377:dbl)
        n212 = local read "User ID"() -> (w386:string)
        n213 = call "DAQ-Abort FGV.vi"("Action"=enum16{"Default", "Init", "Abort", "1st error"}."Init") -> ("Errors"=w384:errorcluster)  [unwired: 12 in, 2 out]
        n214 = control-ref of="SPL History"() -> (w361:refnum<vi>)
        n215 = Unbundle(w388) -> (w387:bool, "Exposure parameters"=w376:T3, "Slack"=w379:T5)
        n216 = call "TB-Config.vi"("Params"=w376, "Exposure?"=w387, "ID"=w386, "error in (no error)"=w384) -> ("state"=w359:T10, "Num Buffers"=w360:i32, "stimulus state"=w363:T13, "StimChan"=w362:T34, "error out"=w381:errorcluster)  [unwired: 7 in]
        n217 = call "TB-Init History.vi"("state"=w359, "Num Buffers"=w360, "XYGraph in"=w361) -> ("history"=w358:cluster{dbl[], dbl[]}[])  [unwired: 12 in]
        n218 = call "TB-Init Logging.vi"("state in"=w359, "Slack"=w379, "Params"=w376, "Level"=w377, "error in (no error)"=w381, "Pistonphone factor"=w368) -> ("Log"=w374:T35, "state out"=w378:T10, "error out"=w380:errorcluster)  [unwired: 7 in]
        n219 = while {
          tunnel: w368 -> [w390]
          tunnel: w360 -> [w416]
          tunnel: w376 -> [w389]
          shift-right: [w418] -> w385
          shift-left: w358 -> [w422]
          shift-right: [w409] -> w382
          shift-left: w380 -> [w408]
          shift-right: [w406] -> w375
          shift-left: w378 -> [w407]
          shift-right: [w404] -> w373
          shift-left: w374 -> [w405]
          shift-right: [w397] -> _
          shift-left: 0 -> [w398]
          shift-right: [w396] -> _
          shift-left: w362 -> [w417]
          shift-right: [w394] -> _
          shift-left: w363 -> [w393]
          tunnel: [w392] -> w369
          tunnel: [w391] -> w367
          stop <- w399 stop-if-true
          n220 = control-ref of="Starts"() -> (w395:refnum<vi>)
          n221 = call "TB-Init Mic Queue.vi"("state in"=w407, "error in (no error)"=w408, "Pistonphone factor"=w390, "Exposure parameters"=w389) -> ("state out"=w402:T10, "mic queue"=w421:T36, "error out"=w403:errorcluster)  [unwired: 9 in]
          n222 = call "TB-Check Initializatin Status.vi"("state in"=w402, "Starts"=w395, "error in (no error)"=w403) -> ("state out"=w401:T10, "error out"=w400:errorcluster)  [unwired: 11 in]
          n223 = Unbundle By Name(w401) -> ("stream mic?"=w413:bool, "stream"=w420:refnum<file>)
          n224 = while {
            tunnel: w416 -> [w452]
            shift-right: [w447] -> w418
            shift-left: w422 -> [w449]
            tunnel: w390 -> [w425]
            tunnel: w389 -> [w433]
            tunnel: w421 -> [w440]
            tunnel: [w440] -> w419
            shift-right: [w429] -> w412
            shift-left: w401 -> [w437]
            tunnel: [w438] -> w415
            shift-right: [w423] -> w397
            shift-left: w398 -> [w434]
            tunnel: [w433] -> w392
            stop <- w439 stop-if-true
            # "# buffers"
            # "SPL History"
            n225 = call "Data Available Queue.vi"() -> ("AI Waveforms"=w443:dbl[][], "error out"=w444:errorcluster)  [unwired: 11 in, 3 out]
            n226 = Unbundle By Name(w433) -> ("Buffer length (s)"=w445:dbl)
            n227 = call "TB-Enqueue Mic Data.vi"("state thru"=w437, "AI Waveforms in"=w443, "error in (no error)"=w444, "Queue in"=w440) -> ("AI Waveforms thru"=w442:dbl[][], "error out"=w441:errorcluster)  [unwired: 10 in]
            n228 = Unbundle By Name(w437) -> ("expose"=w436:bool)
            n229 = call "TB-Analyze.vi"("state in"=w437, "AI Waveforms"=w442, "error in (no error)"=w441, "Exposure parameters"=w433, "Pistonphone Factor"=w425) -> ("state out"=w430:T10, "waveform"=→"Waveform":waveform(dbl), "spectrum"=→"Spectrum":waveform(dbl), "Overload"=→"Overload 2":bool, "Cal SPL"=w427:dbl, "history values"=w424:dbl[], "error out"=w432:errorcluster)  [unwired: 4 in]
            "Gauge" <- w427
            "dB SPL rms" <- w427
            n230 = Increment(x=w434) -> (x+1=w423:i32)
            n231 = Multiply(x=w445, y=w423) -> (x*y=w450:dbl)
            n232 = case shown="True" w436 {
              tunnel: w450 -> [_ w454]
              tunnel: w449 -> [w453 w460]
              tunnel: [w453 w459] -> w447
              tunnel: w424 -> [_ w458]
              tunnel: w423 -> [_ w457]
              frame False {
              }
              frame True {
                n233 = Decrement(x=w457) -> (x-1=w456:i32)
                n234 = Divide(x=w454, y=60.0) -> (x/y=w455:dbl)
                n235 = call "MinSec String.vi"("Seconds"=w454) -> ("MinSec string"=→"Elapsed time":string)
                n236 = call "TB-Update History.vi"("history in"=w460, "history values"=w458, "Index"=w456, "Time"=w455) -> ("history out"=w459:cluster{dbl[], dbl[]}[])  [unwired: 11 in]
              }
            }
            "SPL History" <- w447
            n237 = local read "Fine Control"() -> (w426:dbl)
            n238 = Equal?(x=w452, y=w423) -> (x = y?=w435:bool)
            n239 = call "TB-Update Moving Average.vi"("state in"=w430, "fine"=w426, "SPL"=w427, "error in (no error)"=w432) -> ("state out"=w429:T10, "moving average"=→"ma":dbl, "error out"=w431:errorcluster)  [unwired: 9 in]
            n240 = call "DAQ-Abort FGV.vi"("Finished"=w435, "error in (no error)"=w431) -> ("Stop"=w439:bool, "Errors"=w438:errorcluster)  [unwired: 11 in, 1 out]
          }
          n241 = while {
            shift-right: [w474] -> w414
            shift-left: w400 -> [w475]
            shift-right: [w469] -> w396
            shift-left: w417 -> [w476]
            shift-right: [w465] -> w394
            shift-left: w393 -> [w477]
            tunnel: ["Fine Control"] -> w391
            i -> [w467]
            stop <- w466 stop-if-true
            n242 = call "TB-Create Stimulus.vi"("StimChan In"=w476, "state"=w477, "error in (no error)"=w475, "Fine adjust (dB)"="Fine Control") -> ("StimChan Out"=w469:T34, "state out"=w465:T13, "Stimulus"=w473:dbl[][], "error out"=w472:errorcluster)  [unwired: 8 in]
            n243 = Unbundle By Name(w465) -> ("AO"=w464:i32[])
            n244 = call "Load Signal Bank 1.0.3 keh.vi"("error in (no error)"=w472, "Input array"=w473, "Active AO Array"=w464) -> ("error out"=w471:errorcluster)  [unwired: 6 in, 2 out]
            n245 = Equal To 0?(x=w467) -> (x = 0?=w468:bool)
            n246 = case shown="True" w468 {
              tunnel: w471 -> [w478 w480]
              tunnel: [w478 w479] -> w470
              frame False {
              }
              frame True {
                n247 = call "StartDAQ notifier.vi"("error in (no error)"=w480) -> ("error out"=w479:errorcluster)  [unwired: 6 in]
              }
            }
            n248 = call "DAQ-Abort FGV.vi"("error in (no error)"=w470) -> ("Stop"=w466:bool, "Errors"=w474:errorcluster)  [unwired: 12 in, 1 out]
          }
          n249 = case shown="True" w413 {
            tunnel: w421 -> [_ w482]
            tunnel: w420 -> [_ w481]
            frame False {
            }
            frame True {
              n250 = while {
                tunnel: w482 -> [w491]
                tunnel: w481 -> [w485]
                stop <- w486 stop-if-true
                n251 = Dequeue Element(queue=w491) -> (queue out=w488:T36, element=w489:cluster{bool, dbl[][]}, error out=w490:errorcluster)  [unwired: 2 in, 1 out]
                n252 = case shown="No Error" w490 {
                  selector: w490 -> [_ w515]
                  tunnel: w489 -> [w505 _]
                  tunnel: [w503 TRUE ("status")] -> w487
                  tunnel: w488 -> [w501 w516]
                  tunnel: w485 -> [w500 w517]
                  tunnel: [w499 w517] -> w484
                  tunnel: [w498 w516] -> w483
                  frame No Error {
                    n253 = Unbundle(w505) -> (w504:bool, w502:dbl[][])
                    n254 = case shown="False" w504 {
                      tunnel: [w510 TRUE ("status")] -> w503
                      tunnel: w502 -> [w507 _]
                      tunnel: w501 -> [w511 w512]
                      tunnel: w500 -> [w509 w513]
                      tunnel: [w509 w513] -> w499
                      tunnel: [w511 w512] -> w498
                      frame False {
                        n255 = To Single Precision Float(number=w507) -> (single precision float=w506:sgl[][])
                        n256 = Write to Binary File(file (use dialog)=w509, data=w506) -> (error out=w508:errorcluster)  [unwired: 4 in, 2 out]
                        n257 = call "DAQ-Abort FGV.vi"("error in (no error)"=w508) -> ("Stop"=w510:bool)  [unwired: 12 in, 2 out]
                      }
                      frame True {
                      }
                    }
                  }
                  frame Error {
                    n258 = call "DAQ-Abort FGV.vi"("error in (no error)"=w515) -> ()  [unwired: 12 in, 3 out]
                  }
                }
                n259 = case shown="True" w487 {
                  selector: w487 -> [w492 w497]
                  tunnel: [w492 w497] -> w486
                  tunnel: w484 -> [_ w494]
                  tunnel: w483 -> [_ w496]
                  tunnel: [_ w495] -> _
                  tunnel: [_ w493] -> _
                  frame False {
                  }
                  frame True {
                    n260 = Close File(refnum=w494) -> (error out=w493:errorcluster)  [unwired: 1 in, 1 out]
                    n261 = Release Queue(queue=w496) -> (error out=w495:errorcluster)  [unwired: 2 in, 2 out]
                  }
                }
              }
            }
          }
          n262 = Merge Errors(w415, w414) -> (w411:errorcluster)
          n263 = call "PXI-StopDAQ.vi"("error in (no error)"=w411) -> ("error out"=w410:errorcluster)  [unwired: 6 in]
          n264 = call "TB-Stop.vi"("state in"=w412, "Log in"=w405, "error in (no error)"=w410, "Queue in"=w419) -> ("Log out"=w404:T35, "state out"=w406:T10, "Finished"=w399:bool, "error out"=w409:errorcluster)  [unwired: 8 in]
        }
        n265 = control-ref of="SPL History"() -> (w370:refnum<vi>)
        n266 = control-ref of="This VI"() -> (w366:refnum<vi>)
        n267 = Unbundle By Name(w375) -> ("expose"=w383:bool)
        n268 = case shown="True" w383 {
          tunnel: w385 -> [_ w536]
          tunnel: w375 -> [w525 w535]
          tunnel: w382 -> [w524 w534]
          tunnel: w373 -> [_ w530]
          tunnel: w370 -> [_ w528]
          tunnel: w369 -> [w526 w527]
          tunnel: w367 -> [w521 _]
          tunnel: w366 -> [w520 _]
          tunnel: [w519 _] -> w365
          tunnel: w364 -> [_ w529]
          frame False {
            n269 = call "TB-Save Setup Log.vi"("State"=w525, "VI ref"=w520, "Exposure parameters"=w526, "Fine Control"=w521) -> ("date/time string"=w519:string, "error out"=w522:errorcluster)  [unwired: 10 in]
            n270 = Merge Errors(w524, w522) -> (w523:errorcluster)
            n271 = property on="Crown" class="Clust (strict)"("Val(Sgnl)"=w523) -> ()  [unwired: 2 in, 2 out]
          }
          frame True {
            n272 = call "TB-Save SPL History.vi"("state"=w535, "Log in"=w530, "XYGraph in"=w528, "date/time string"=w529, "history"=w536, "Exposure parameters"=w527) -> ("error out"=w532:errorcluster)  [unwired: 9 in]
            n273 = call "TB-Slack Figure.vi"("Log"=w530, "XYGraph in"=w528) -> ("error out"=w531:errorcluster)  [unwired: 13 in]
            n274 = Merge Errors(w534, w532, w531) -> (w533:errorcluster)
            n275 = property on="Exposure" class="Clust (strict)"("Val(Sgnl)"=w533) -> ()  [unwired: 2 in, 2 out]
          }
        }
      }
      frame Error {
      }
    }
  }
  n276 = disable-structure shown="RUN_TIME_ENGINE==True" {
    disable-tunnel: w7 -> [w537 _]
    frame condition #0 {
      n277 = Quit LabVIEW(quit? (T)=w537) -> ()
    }
    frame condition #1 (active) {
    }
  }
